vi "Calibration-Frame14.vi"(10 "Results file output":path, 11 "String":string) -> ()   [LabVIEW 2015]
uses:
  Anemometry Sub Vis/Globals/Calib_global.vi
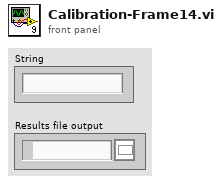
[diagram p1: front panel]
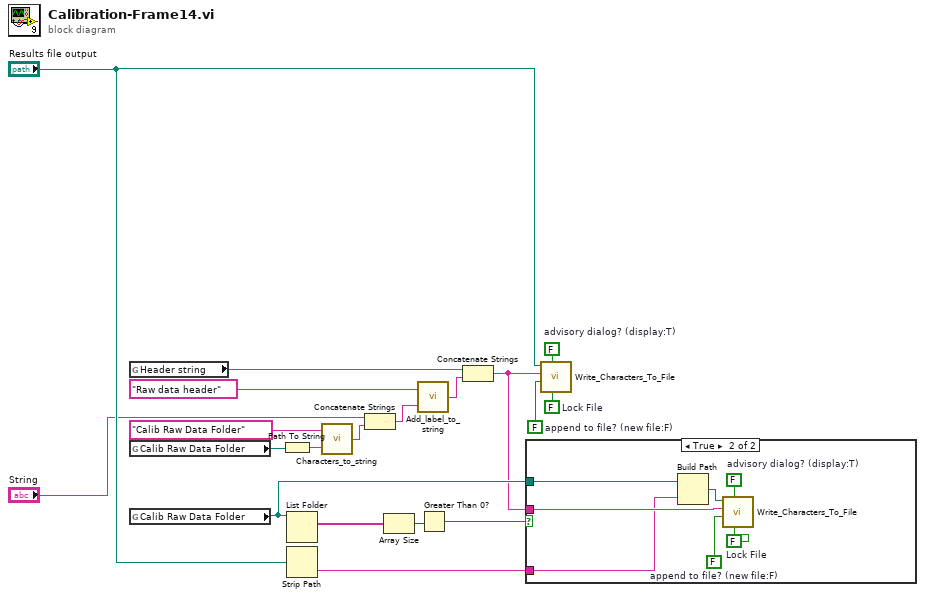
[diagram p0: block diagram]
diagram:
  w4 = FALSE  # Lock File
  w2 = FALSE  # advisory dialog? (display:T)
  w1 = FALSE  # append to file? (new file:F)
  n1 = global read "Calib_global.vi" "Header string"() -> (w3:string)
  n2 = global read "Calib_global.vi" "Calib Raw Data Folder"() -> (w11:path)
  n3 = global read "Calib_global.vi" "Calib Raw Data Folder"() -> (w10:path)
  n4 = Path To String(path=w11) -> (string=w12:string)
  n5 = List Folder(path=w10) -> (filenames=w7:string[])  [unwired: 1 in, 5 out]
  n6 = Strip Path(path="Results file output") -> (name=w6:string)  [unwired: 1 out]
  n7 = call "Characters_to_string.vi"("Characters to write"=w12, "Label for characters"="Calib Raw Data Folder") -> ("Output string"=w15:string)
  n8 = Concatenate Strings("String", w15) -> (w16:string)
  n9 = Array Size(array=w7) -> (size(s)=w8:i32)
  n10 = call "Add_label_to_string.vi"("String to write"=w16, "File Label"="Raw data header") -> ("Output string"=w18:string)
  n11 = Greater Than 0?(x=w8) -> (x > 0?=w9:bool)
  n12 = Concatenate Strings(w3, w18) -> (w5:string)
  n13 = case shown="True" w9 {
    tunnel: w5 -> [_ w23]
    tunnel: w6 -> [_ w22]
    tunnel: w10 -> [_ w20]
    frame False {
    }
    frame True {
      w24 = FALSE  # Lock File
      w25 = FALSE  # append to file? (new file:F)
      w26 = FALSE  # advisory dialog? (display:T)
      n14 = Build Path(base path=w20, name or relative path=w22) -> (appended path=w21:path)
      n15 = call "Write_Characters_To_File.vi"("file path (dialog if empty)"=w21, "advisory dialog? (display:T)"=w26, "character string"=w23, "append to file? (new file:F)"=w25, "Lock File"=w24) -> ()  [unwired: 4 out]
    }
  }
  n16 = call "Write_Characters_To_File.vi"("file path (dialog if empty)"="Results file output", "advisory dialog? (display:T)"=w2, "character string"=w5, "append to file? (new file:F)"=w1, "Lock File"=w4) -> ()  [unwired: 4 out]
